vi "Boolean Shooting Dice.vi"() -> ()   [LabVIEW 2019]
uses:
  <vilib>/numeric/Random Number (Range) U64.vi
  <vilib>/numeric/sub_Random U32.vi
panel:
  out "Snake Eyes":bool
  out "Dice Total:":dbl
  out "Second Die:":dbl
  in  "Press to roll the dice":bool
  out "First Die:":dbl
  # "Challenge:\nShooting Dice. When the button is pressed, two dice are rolled. The value of each die is displayed, along with the total of the two dice. An LED lights up if Snake Eyes (two ones) is rolled. Note: You can use the Roll of the Die challenge program to help you get started."
  # "Try it: Run the program and press the button to roll the dice."
  # "You will probably need:\nBooleans, random number generator, front panel control, numeric functions"
  # "Open the block diagram to see a possible solution."
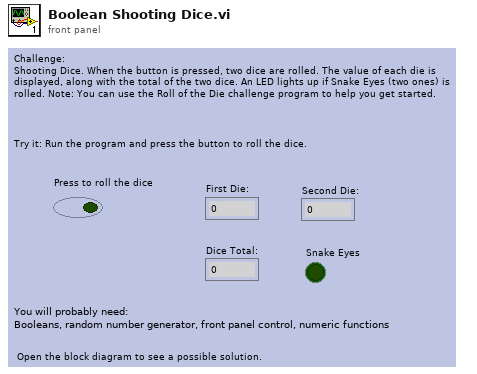
[diagram p1: front panel]
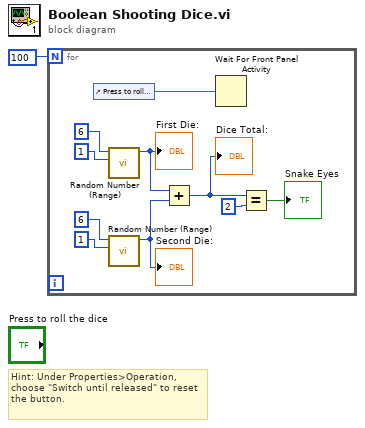
[diagram p0: block diagram]
diagram:
  # "Hint: Under Properties>Operation, choose \"Switch until released\" to reset the button."
  n1 = for {
    N: 100 -> [_]
    n2 = control-ref of="Press to roll the dice"() -> (w9:refnum<vi>)
    n3 = call-poly <vilib>:"Random Number (Range).vi"("lower bound (0)"=u64 1, "upper bound (100)"=u64 6) -> ("number"=w6:u64)  [unwired: 9 in]
    "First Die:" <- w6
    n4 = call-poly <vilib>:"Random Number (Range).vi"("lower bound (0)"=u64 1, "upper bound (100)"=u64 6) -> ("number"=w5:u64)  [unwired: 9 in]
    "Second Die:" <- w5
    n5 = Add(x=w6, y=w5) -> (x+y=w4:u64)
    "Dice Total:" <- w4
    n6 = Wait For Front Panel Activity(2:w9) -> ()  [unwired: 2 in, 1 out]
    n7 = Equal?(x=w4, y=2) -> (x = y?=→"Snake Eyes":bool)
  }
